vi "MCL Get All Handles.vi"(8 "error in (no error)":errorcluster, 10 "size":i32, 11 "handles":i32) -> (0 "error out":errorcluster, 2 "function return":i32, 3 "handles out":i32)   [LabVIEW 2014, in "Madlib.lvlib"]
doc: "MADLIB_API int MCL_GetAllHandles(int *handles, int size);"
uses:
  <userlib>/Lambda2/lib/Madlib/Madlib.lvlib
  <userlib>/Lambda2/lib/Madlib/Madlib.dll
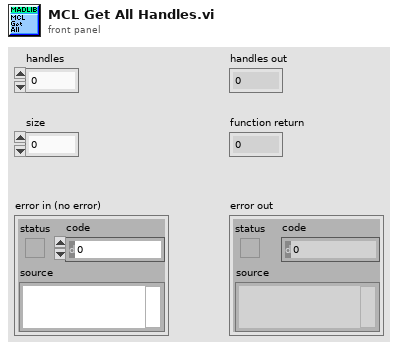
[diagram p1: front panel]
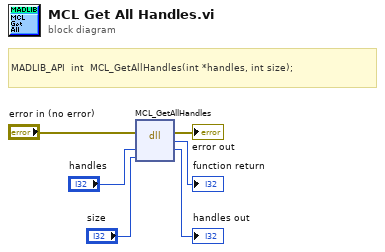
[diagram p0: block diagram]
diagram:
  # "MADLIB_API  int\t\tMCL_GetAllHandles(int *handles, int size);"
  n1 = dll-call lib="C:/Program Files (x86)/National Instruments/LabVIEW 2014/user.lib/Lambda2/lib/Madlib/Madlib.*" fn="MCL_GetAllHandles"(error in="error in (no error)", "handles"="handles", "size"="size") -> (error out=→"error out":errorcluster, →"function return":i32, "handles"=→"handles out":i32)  [unwired: 3 in, 1 out]
